vi "CRYChannel num to string.vi"(11 "Channel":i32) -> (3 "Channel string":string)   [LabVIEW 2013]
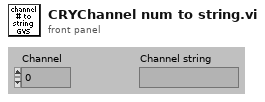
[diagram p1: front panel]
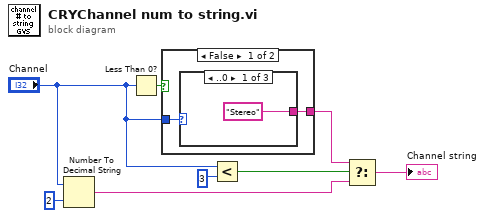
[diagram p0: block diagram]
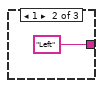
[diagram p2: hidden frame]
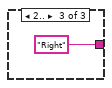
[diagram p3: hidden frame]
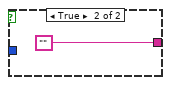
[diagram p4: hidden frame]
diagram:
  n1 = Number To Decimal String(number="Channel", width (-)=i16 2) -> (decimal integer string=w8:string)
  n2 = Less Than 0?(x="Channel") -> (x < 0?=w5:bool)
  n3 = case shown="False" w5 {
    tunnel: "Channel" -> [w10 _]
    tunnel: [w9 ""] -> w4
    frame False {
      n4 = case shown="..0" w10 {
        tunnel: ["Stereo" "Left" "Right"] -> w9
        frame ..0 {
        }
        frame 1 {
        }
        frame 2.. {
        }
      }
    }
    frame True {
    }
  }
  n5 = Less?(x="Channel", y=3) -> (x < y?=w2:bool)
  n6 = Select(t=w4, s=w2, f=w8) -> (s? t:f=→"Channel string":string)
